vi "remove_invalid_ROI.vi"(8 "error in (no error)":errorcluster, 9 "number of particles":i32, 10 "Image Pixels in":u8[][](array[numeric]), 11 "SegmenterMG100305SingleCell in":refnum<class "SegmenterMG100305SingleCell.lvclass">) -> (0 "error out":errorcluster, 1 "ROI array out":cluster{"x":i32, "y":i32}[](array[cluster]), 2 "Image Pixels out":u8[][](array[numeric]), 3 "SegmenterMG100305SingleCell out":refnum<class "SegmenterMG100305SingleCell.lvclass">)   [LabVIEW 2010, in "SegmenterMG100305SingleCell.lvclass"]
uses:
  SegmenterMG100305SingleCell.lvclass
  <vilib>/Analysis/Matrix/Datatypes/RealMatrix.ctl
  <vilib>/Analysis/Matrix/NI_Matrix.lvlib
panel:
  out "Real Matrix":T1
  out "Numeric":i32
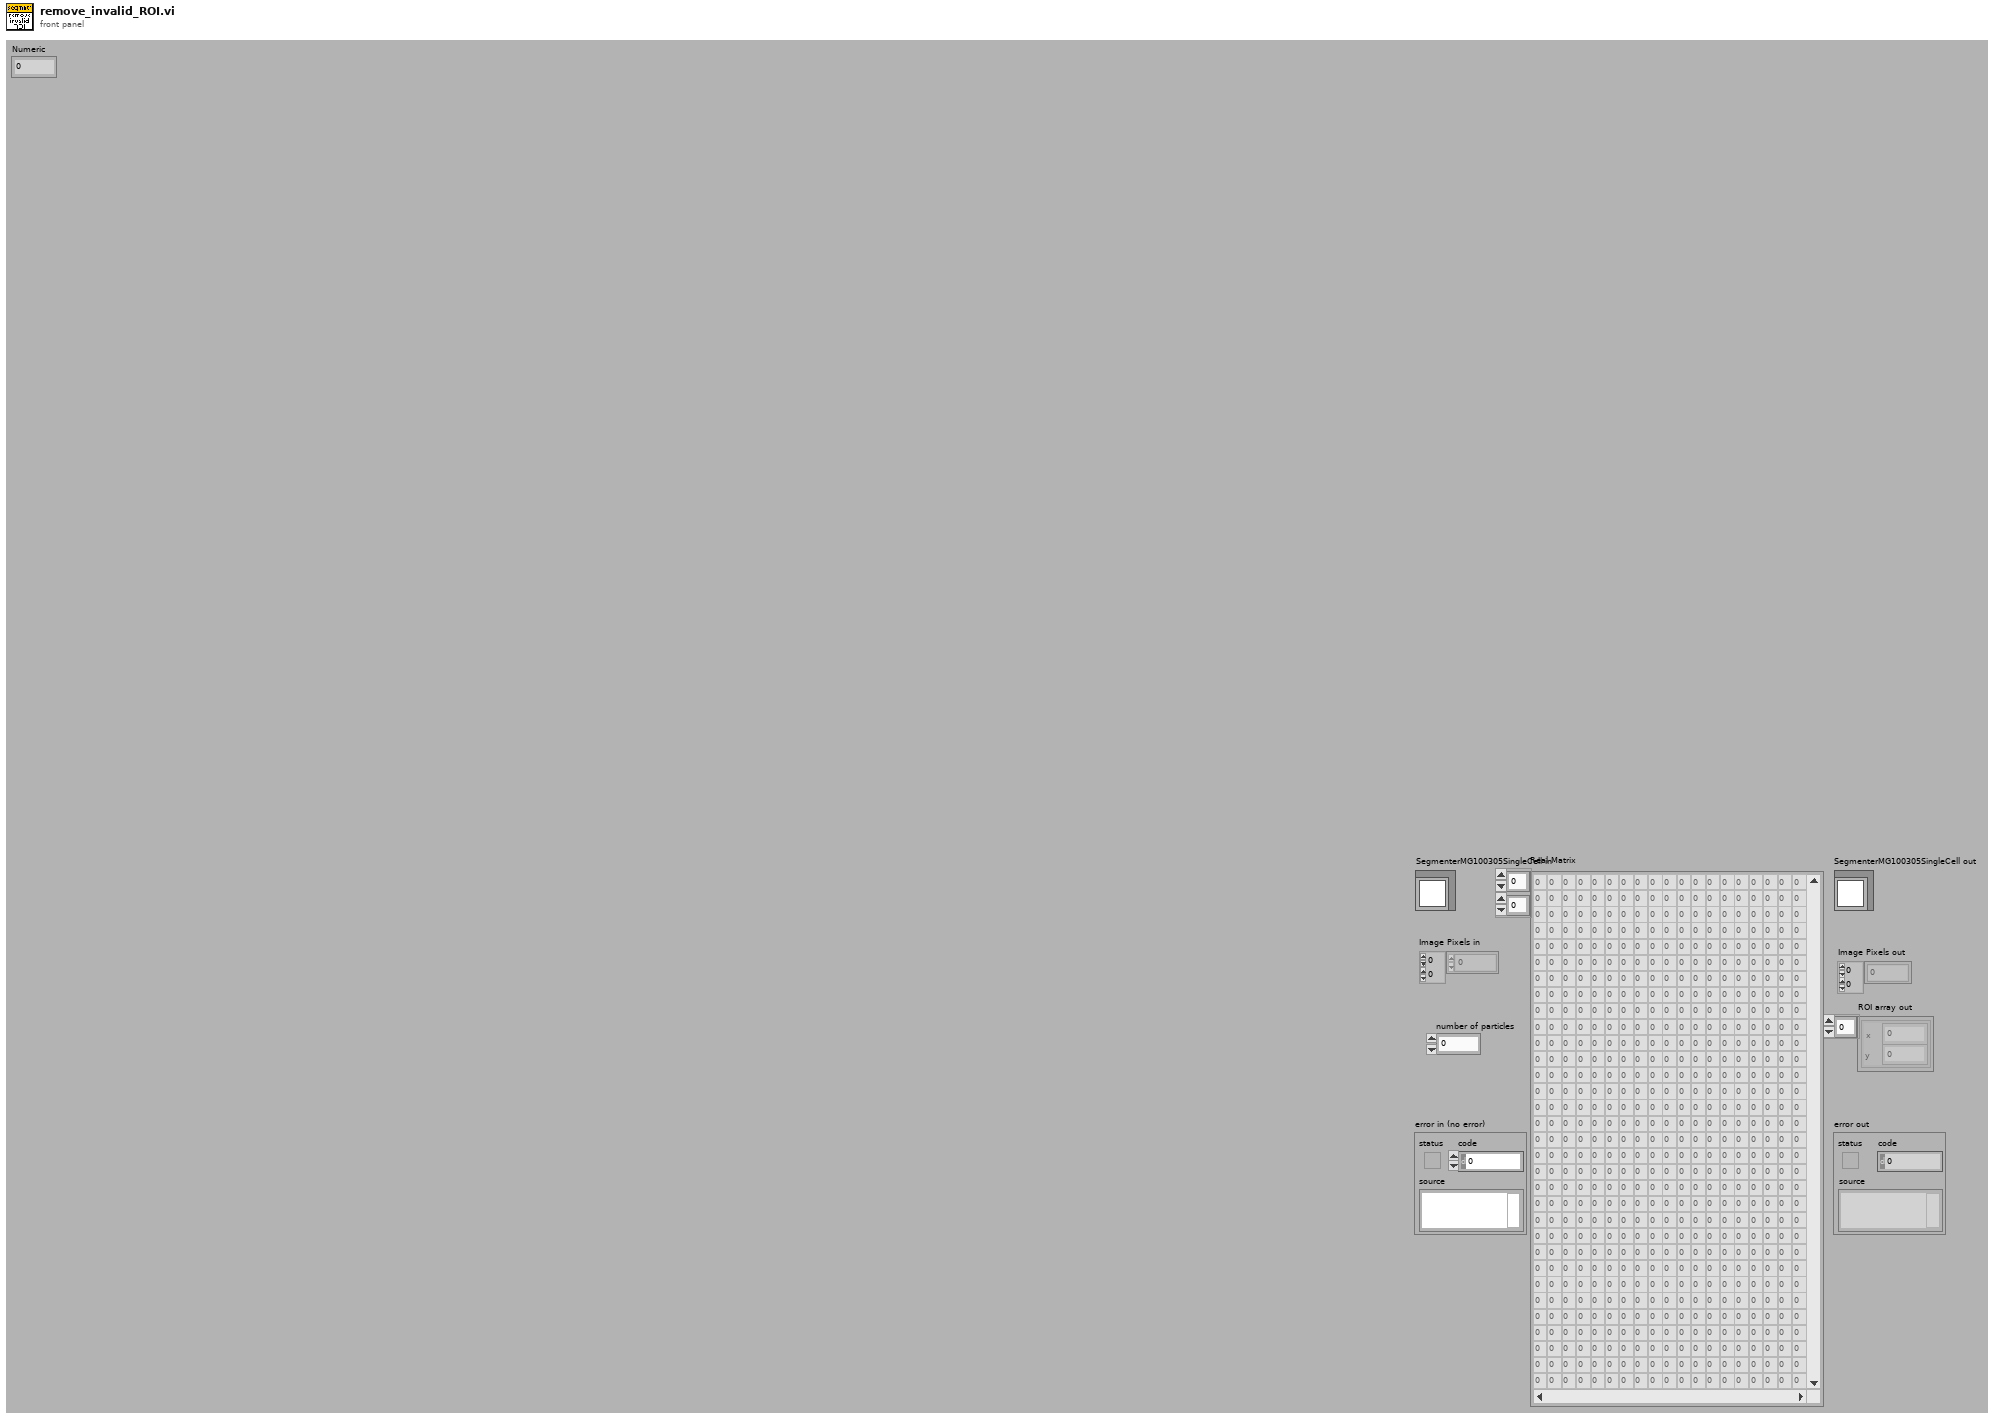
[diagram p1: front panel]
types:
  T1 = typedef "NI_Matrix.lvlib/RealMatrix.ctl" = dbl[][]
  T2 = cluster{"[0]":i32, "[1]":i32, "[2]":i32, "[3]":i32, "[4]":i32, "[5]":i32, "[6]":i32, "[7]":i32, "[8]":i32}
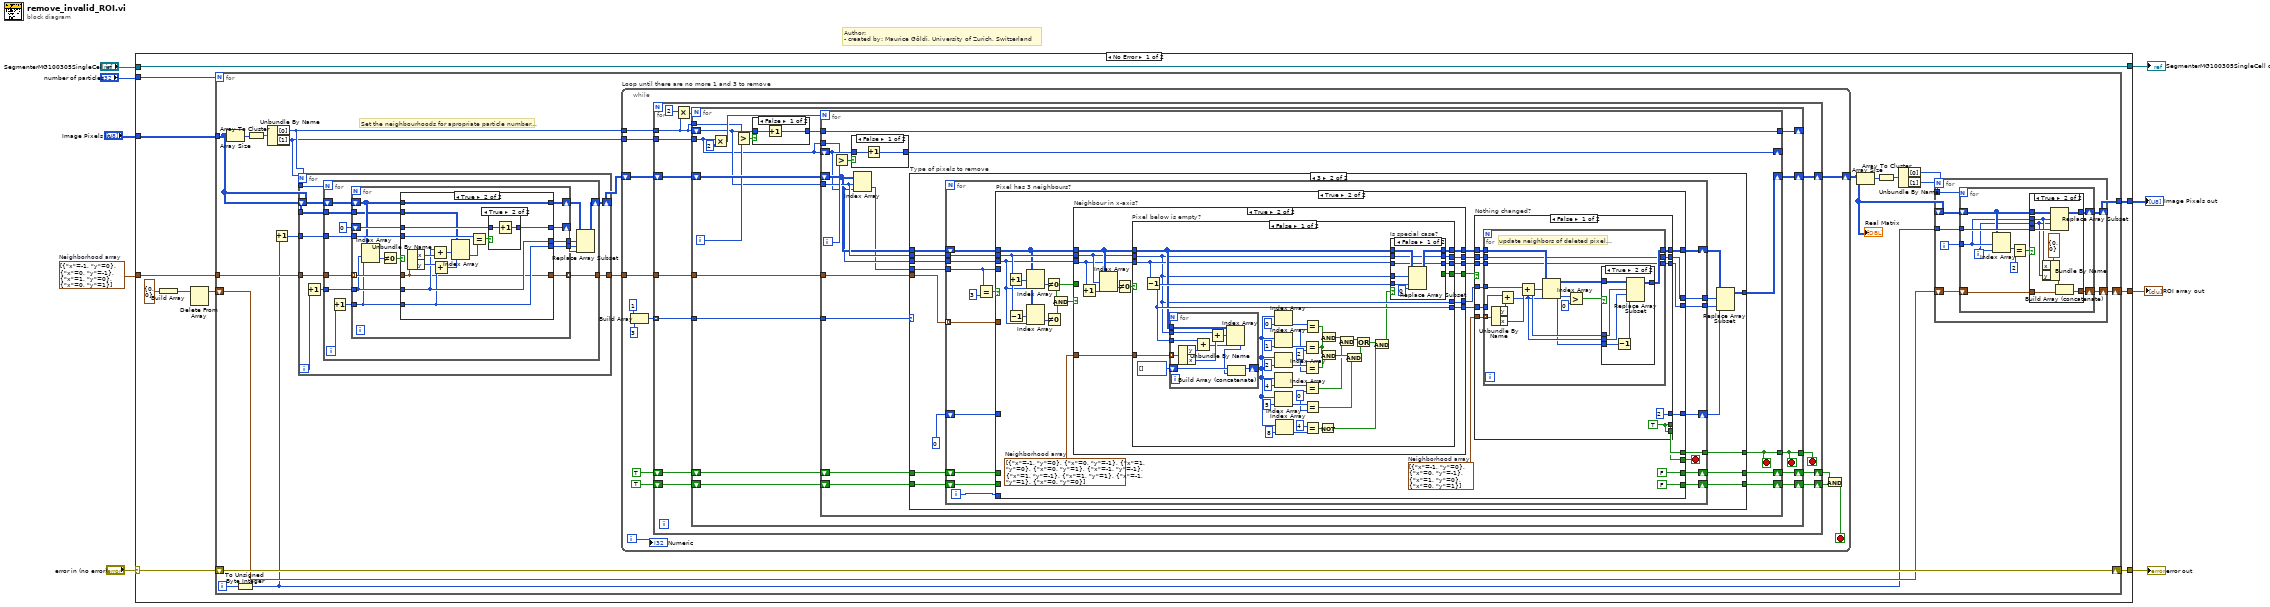
[diagram p0: block diagram]
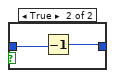
[diagram p5: hidden frame]
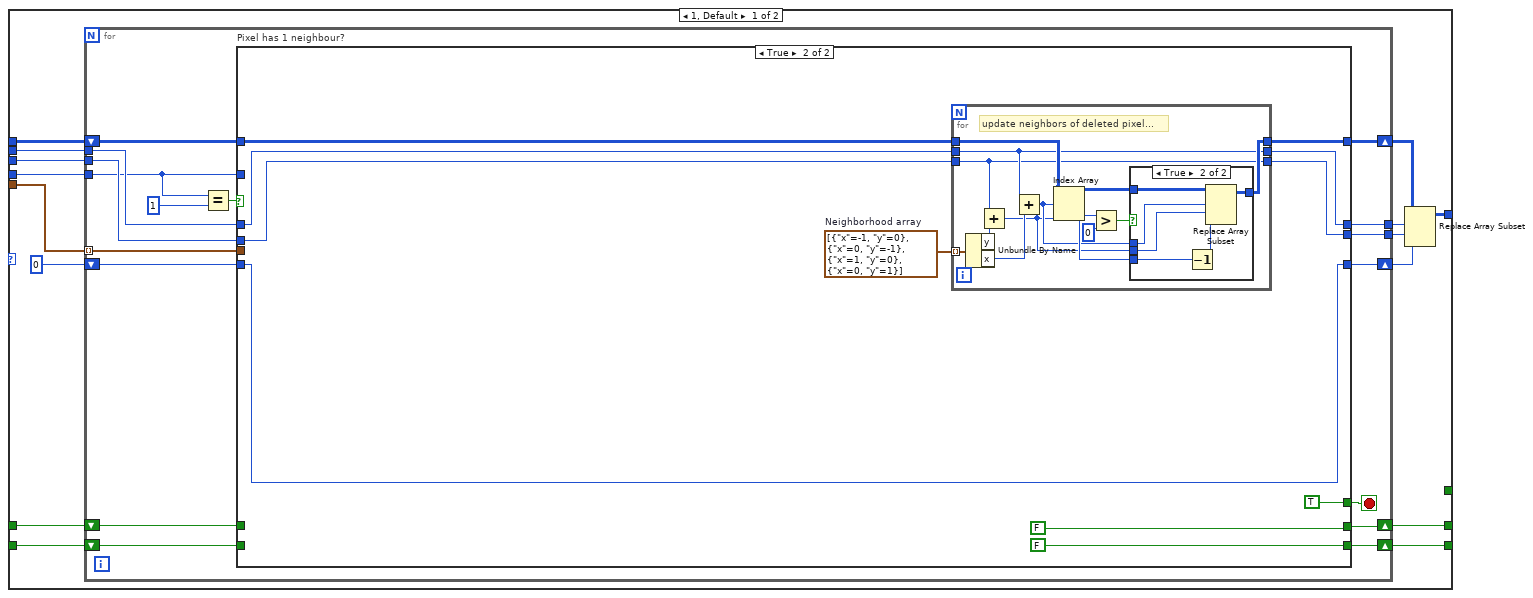
[diagram p6: hidden frame]
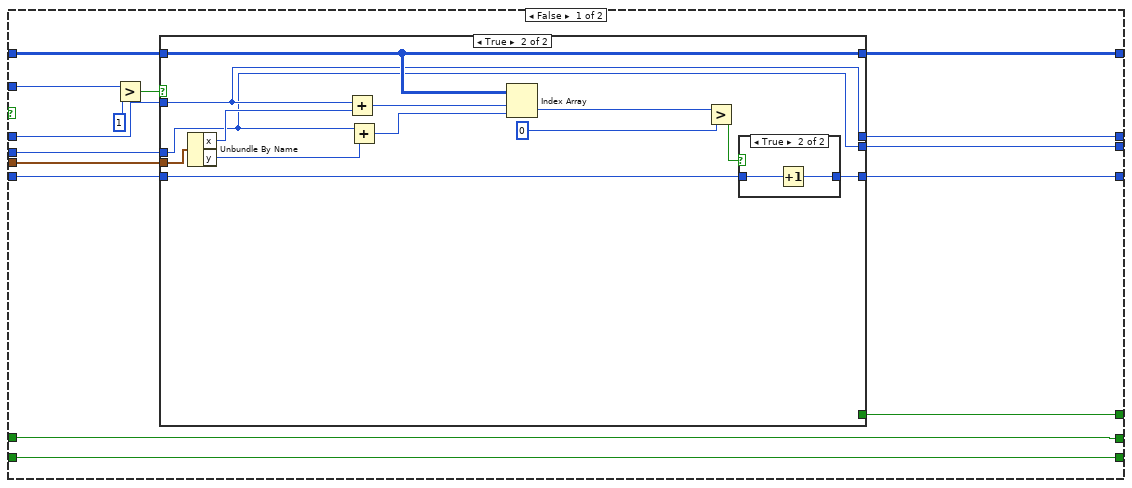
[diagram p7: hidden frame]
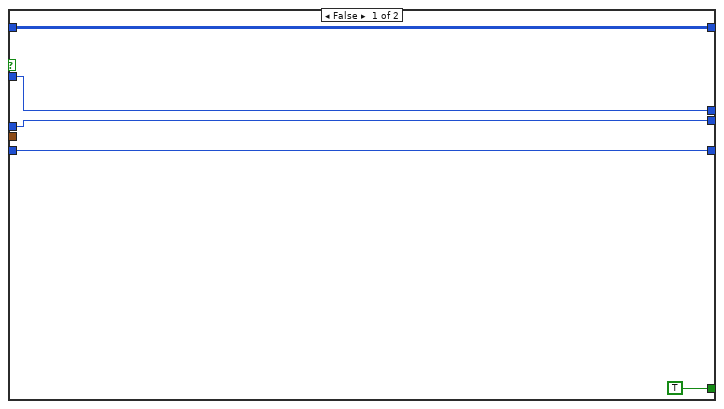
[diagram p8: hidden frame]
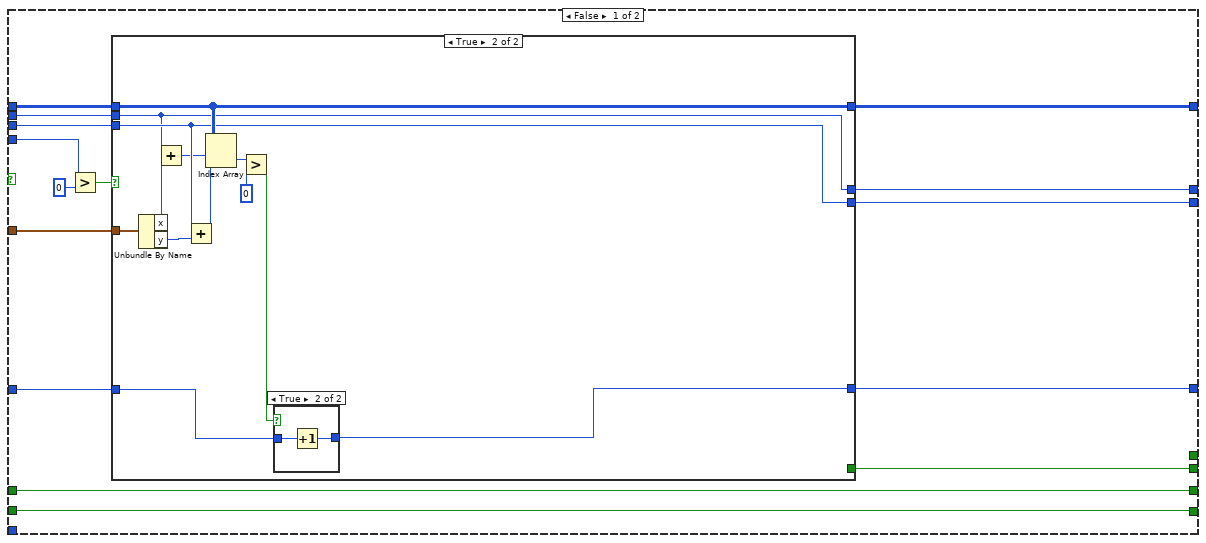
[diagram p11: hidden frame]
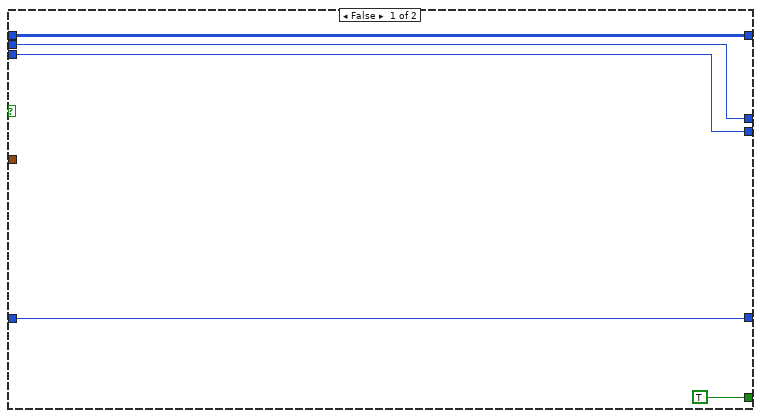
[diagram p12: hidden frame]
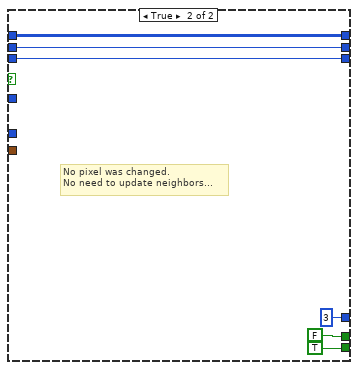
[diagram p15: hidden frame]
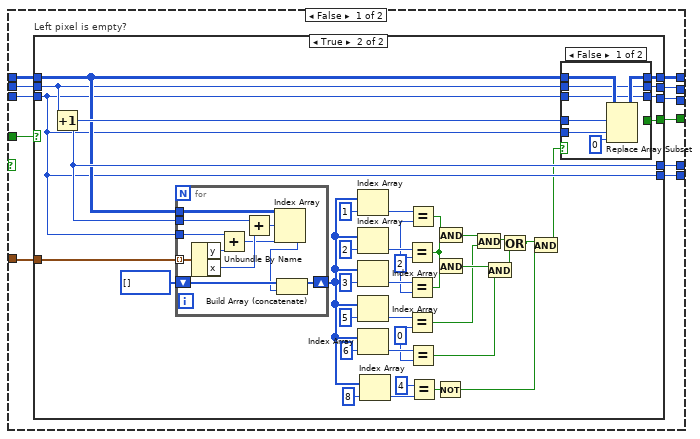
[diagram p16: hidden frame]
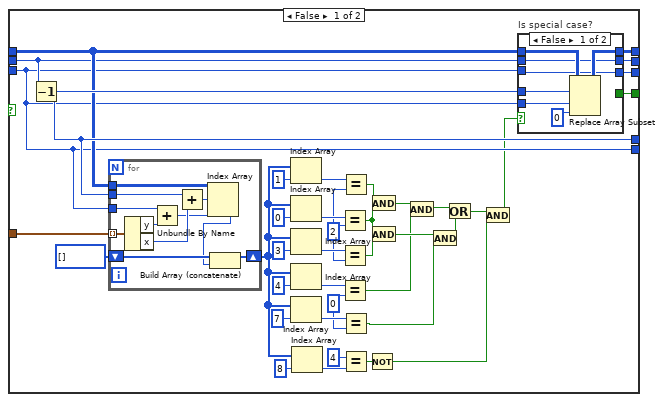
[diagram p17: hidden frame]
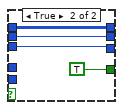
[diagram p18: hidden frame]
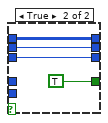
[diagram p19: hidden frame]
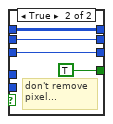
[diagram p20: hidden frame]
diagram:
  w5 = cluster{"x":i32, "y":i32}[] [{"x"=-1, "y"=0}, {"x"=0, "y"=-1}, {"x"=1, "y"=0}, {"x"=0, "y"=1}]  # Neighborhood array
  # "Author: \n- created by: Maurice Göldi, University of Zurich, Switzerland"
  n1 = case shown="No Error" "error in (no error)" {
    selector: "error in (no error)" -> [w17 w700]
    tunnel: [w16 w700] -> w6
    tunnel: "number of particles" -> [w20 _]
    tunnel: "Image Pixels in" -> [w19 _]
    tunnel: w5 -> [w18 _]
    tunnel: [w15 _] -> w1
    tunnel: [w14 _] -> w2
    tunnel: "SegmenterMG100305SingleCell in" -> [w11 w699]
    tunnel: [w11 w699] -> w7
    frame No Error {
      n2 = Build Array(cluster{"x":i32, "y":i32} {"x"=0, "y"=0} ("point")) -> (w13:cluster{"x":i32, "y":i32}[])
      n3 = Delete From Array(array=w13) -> (array with subset deleted=w12:cluster{"x":i32, "y":i32}[])  [unwired: 2 in, 1 out]
      n4 = for {
        N: w20 -> [_]
        tunnel: w19 -> [w22]
        tunnel: w18 -> [w35]
        shift-right: [w40] -> w16
        shift-left: w17 -> [w40]
        shift-right: [w28] -> w15
        shift-left: w12 -> [w27]
        tunnel: [w26] -> w14
        i -> [w25]
        # "Set the neighbourhoods for apropriate particle number..."
        n5 = Array Size(array=w22) -> (size(s)=w39:i32[])
        n6 = To Unsigned Byte Integer(number=w25) -> (unsigned 8bit integer=w24:u8)
        n7 = Array To Cluster(array=w39) -> (cluster=w38:T2)
        n8 = Unbundle By Name(w38) -> ("[0]"=w37:i32, "[1]"=w36:i32)
        n9 = Increment(x=w24) -> (x+1=w33:u8)
        n10 = for {
          N: w37 -> [_]
          tunnel: w36 -> [w77]
          shift-right: [w75] -> w23
          shift-left: w22 -> [w76]
          tunnel: w35 -> [w74]
          tunnel: [w73] -> w34
          tunnel: w33 -> [w70]
          tunnel: w22 -> [w69]
          i -> [w72]
          n11 = Increment(x=w72) -> (x+1=w71:i32)
          n12 = for {
            N: w77 -> [_]
            shift-right: [w82] -> w75
            shift-left: w76 -> [w89]
            tunnel: [w91] -> w73
            tunnel: w74 -> [w90]
            tunnel: w71 -> [w87]
            tunnel: w70 -> [w85]
            tunnel: w69 -> [w78]
            i -> [w88]
            n13 = Increment(x=w88) -> (x+1=w86:i32)
            n14 = for {
              tunnel: [w93] -> w91 mode=indexing
              tunnel: w90 -> [w105] mode=indexing
              shift-right: [w100] -> w83
              shift-left: w89 -> [w98]
              tunnel: w87 -> [w97]
              tunnel: w86 -> [w96]
              tunnel: w85 -> [w99]
              shift-right: [w103] -> w81
              shift-left: u8 0 -> [w104]
              tunnel: [w102] -> w80
              tunnel: [w101] -> w79
              tunnel: w78 -> [w92]
              n15 = Index Array(array=w98, index (row)=w97, index (col)=w96) -> (element=w94:u8)
              n16 = Not Equal To 0?(x=w94) -> (x != 0?=w95:bool)
              n17 = case shown="True" w95 {
                tunnel: w105 -> [w106 w112]
                tunnel: w98 -> [w107 w113]
                tunnel: w99 -> [_ w118]
                tunnel: w104 -> [w108 w117]
                tunnel: [w108 w116] -> w103
                tunnel: w96 -> [w109 w114]
                tunnel: w97 -> [w110 w115]
                tunnel: [w110 w115] -> w102
                tunnel: [w109 w114] -> w101
                tunnel: [w107 w113] -> w100
                tunnel: [w106 w112] -> w93
                tunnel: w92 -> [_ w111]
                frame False {
                }
                frame True {
                  n18 = Unbundle By Name(w112) -> ("x"=w124:i32, "y"=w123:i32)
                  n19 = Add(x=w115, y=w124) -> (x+y=w122:i32)
                  n20 = Add(x=w123, y=w114) -> (x+y=w121:i32)
                  n21 = Index Array(array=w111, index (row)=w122, index (col)=w121) -> (element=w119:u8)
                  n22 = Equal?(x=w118, y=w119) -> (x = y?=w120:bool)
                  n23 = case shown="True" w120 {
                    tunnel: [w125 w127] -> w116
                    tunnel: w117 -> [w125 w126]
                    frame False {
                    }
                    frame True {
                      n24 = Increment(x=w126) -> (x+1=w127:u8)
                    }
                  }
                }
              }
            }
            n25 = Replace Array Subset(array=w83, new element=w81, index (row)=w80, index (col)=w79) -> (w82:u8[][])
          }
        }
        n26 = while "Loop until there are no more 1 and 3 to remove" {
          tunnel: w34 -> [w141]
          tunnel: w37 -> [w136]
          tunnel: w36 -> [w135]
          shift-right: [w134] -> w21
          shift-left: w23 -> [w133]
          i -> [w132]
          stop <- w130 stop-if-true
          n27 = Build Array(1 ("element"), 3 ("element")) -> (w138:i32[])
          n28 = for {
            tunnel: w141 -> [w151]
            tunnel: w138 -> [w150] mode=indexing
            tunnel: w136 -> [w146]
            tunnel: w135 -> [w148]
            shift-right: [w147] -> w134
            shift-left: w133 -> [w154]
            shift-right: [w143] -> w129
            shift-left: TRUE -> [w149]
            shift-right: [w144] -> w128
            shift-left: TRUE -> [w145]
            stop <- w142 stop-if-true
            n29 = Multiply(x=2, y=w146) -> (x*y=w153:i32)
            n30 = for {
              N: w153 -> [_]
              tunnel: w148 -> [w158]
              shift-right: [w170] -> _
              shift-left: w146 -> [w164]
              shift-right: [w168] -> w147
              shift-left: w154 -> [w169]
              tunnel: w151 -> [w163]
              tunnel: w150 -> [w162]
              shift-right: [w160] -> w143
              shift-left: w149 -> [w161]
              tunnel: w146 -> [w159]
              shift-right: [w156] -> w144
              shift-left: w145 -> [w157]
              tunnel: [w155] -> w142
              i -> [w165]
              stop <- w155 stop-if-true
              n31 = Multiply(x=w158, y=2) -> (x*y=w171:i32)
              n32 = Greater?(x=w159, y=w165) -> (0:w166:bool)
              n33 = case shown="False" w166 {
                tunnel: w164 -> [w174 w175]
                tunnel: [w173 w176] -> w167
                frame False {
                  n34 = Increment(x=w174) -> (x+1=w173:i32)
                }
                frame True {
                  n35 = Decrement(x=w175) -> (x-1=w176:i32)
                }
              }
              n36 = for {
                N: w171 -> [_]
                shift-right: [w192] -> _
                shift-left: w158 -> [w185]
                shift-right: [w183] -> w168
                shift-left: w169 -> [w186]
                tunnel: w164 -> [w187]
                tunnel: w163 -> [w189]
                tunnel: w162 -> [w188]
                shift-right: [w181] -> w160
                shift-left: w161 -> [w182]
                tunnel: w158 -> [w180]
                shift-right: [w178] -> w156
                shift-left: w157 -> [w179]
                tunnel: w167 -> [w193]
                tunnel: [w193] -> w170
                tunnel: [w177] -> w155
                i -> [w190]
                stop <- w177 stop-if-true
                n37 = Greater?(x=w180, y=w190) -> (0:w191:bool)
                n38 = case shown="False" w191 {
                  tunnel: w185 -> [w696 w697]
                  tunnel: [w695 w698] -> w192
                  frame False {
                    n39 = Increment(x=w696) -> (x+1=w695:i32)
                  }
                  frame True {
                    n40 = Decrement(x=w697) -> (x-1=w698:i32)
                  }
                }
                n41 = Index Array(array=w186, index (row)=w187, index (col)=w185) -> (element=w184:u8)
                n42 = case "Type of pixels to remove" shown="3" w188 {
                  tunnel: w189 -> [w208 w303]
                  tunnel: w187 -> [w207 w306]
                  tunnel: w185 -> [w206 w305]
                  tunnel: w186 -> [w205 w307]
                  tunnel: w184 -> [w204 w304]
                  tunnel: [w198 w301] -> w183
                  tunnel: w182 -> [w196 w297]
                  tunnel: [w195 w296] -> w181
                  tunnel: w179 -> [w197 w294]
                  tunnel: [w194 w293] -> w178
                  tunnel: [_ w292] -> w177
                  frame 1, Default {
                    n43 = for {
                      tunnel: w208 -> [w219] mode=indexing
                      tunnel: w207 -> [w223]
                      tunnel: w206 -> [w222]
                      shift-right: [w216] -> w201
                      shift-left: w205 -> [w220]
                      tunnel: w204 -> [w221]
                      shift-right: [w217] -> w202
                      shift-left: u8 0 -> [w218]
                      tunnel: [w215] -> w200
                      tunnel: [w214] -> w199
                      shift-right: [w212] -> w194
                      shift-left: w197 -> [w211]
                      shift-right: [w209] -> w195
                      shift-left: w196 -> [w210]
                      stop <- w213 stop-if-true
                      n44 = Equal?(x=w221, y=u8 1) -> (x = y?=w224:bool)
                      n45 = case "Pixel has 1 neighbour?" shown="True" w224 {
                        tunnel: w220 -> [w232 w268]
                        tunnel: w223 -> [w236 w266]
                        tunnel: w222 -> [w235 w265]
                        tunnel: w221 -> [w239 _]
                        tunnel: w219 -> [w237 _]
                        tunnel: w218 -> [w234 w264]
                        tunnel: [w233 w264] -> w217
                        tunnel: [w231 w269] -> w216
                        tunnel: [w230 w263] -> w215
                        tunnel: [w229 w262] -> w214
                        tunnel: [w228 TRUE] -> w213
                        tunnel: [w226 FALSE] -> w212
                        tunnel: w211 -> [w226 _]
                        tunnel: [w227 FALSE] -> w209
                        tunnel: w210 -> [w227 _]
                        frame False {
                          n46 = Greater?(x=w239, y=u8 1) -> (0:w240:bool)
                          n47 = case shown="True" w240 {
                            tunnel: w232 -> [w244 w250]
                            tunnel: w237 -> [_ w256]
                            tunnel: w236 -> [w243 w249]
                            tunnel: w235 -> [w242 w248]
                            tunnel: w234 -> [w245 w252]
                            tunnel: [w245 w251] -> w233
                            tunnel: [w244 w250] -> w231
                            tunnel: [w243 w249] -> w230
                            tunnel: [w242 w248] -> w229
                            tunnel: [TRUE _] -> w228
                            frame False {
                            }
                            frame True {
                              n48 = Unbundle By Name(w256) -> ("x"=w257:i32, "y"=w258:i32)
                              n49 = Add(x=w249, y=w257) -> (x+y=w247:i32)
                              n50 = Add(x=w248, y=w258) -> (x+y=w246:i32)
                              n51 = Index Array(array=w250, index (row)=w247, index (col)=w246) -> (element=w255:u8)
                              n52 = Greater?(x=w255, y=u8 0) -> (0:w253:bool)
                              n53 = case shown="True" w253 {
                                tunnel: w252 -> [w259 w261]
                                tunnel: [w259 w260] -> w251
                                frame False {
                                }
                                frame True {
                                n54 = Increment(x=w261) -> (x+1=w260:u8)
                                }
                              }
                            }
                          }
                        }
                        frame True {
                          w267 = cluster{"x":i32, "y":i32}[] [{"x"=-1, "y"=0}, {"x"=0, "y"=-1}, {"x"=1, "y"=0}, {"x"=0, "y"=1}]  # Neighborhood array
                          n55 = for {
                            tunnel: w267 -> [w284] mode=indexing
                            tunnel: w265 -> [w273]
                            tunnel: w266 -> [w274]
                            tunnel: [w283] -> w269
                            tunnel: w268 -> [w282]
                            tunnel: [w274] -> w263
                            tunnel: [w273] -> w262
                            # "update neighbors of deleted pixel..."
                            n56 = Unbundle By Name(w284) -> ("y"=w281:i32, "x"=w280:i32)
                            n57 = Add(x=w273, y=w281) -> (x+y=w275:i32)
                            n58 = Add(x=w274, y=w280) -> (x+y=w276:i32)
                            n59 = Index Array(array=w282, index (row)=w276, index (col)=w275) -> (element=w277:u8)
                            n60 = Greater?(x=w277, y=u8 0) -> (0:w279:bool)
                            n61 = case shown="True" w279 {
                              tunnel: [w285 w291] -> w283
                              tunnel: w282 -> [w285 w290]
                              tunnel: w277 -> [_ w287]
                              tunnel: w276 -> [_ w289]
                              tunnel: w275 -> [_ w288]
                              frame False {
                              }
                              frame True {
                                n62 = Decrement(x=w287) -> (x-1=w286:u8)
                                n63 = Replace Array Subset(array=w290, new element=w286, index (row)=w289, index (col)=w288) -> (w291:u8[][])
                              }
                            }
                          }
                        }
                      }
                    }
                    n64 = Replace Array Subset(array=w201, new element=w202, index (row)=w200, index (col)=w199) -> (w198:u8[][])
                  }
                  frame 3 {
                    n65 = for {
                      tunnel: w306 -> [w323]
                      tunnel: w305 -> [w322]
                      tunnel: w304 -> [w314]
                      tunnel: w303 -> [w321] mode=indexing
                      shift-right: [w318] -> w295
                      shift-left: w307 -> [w326]
                      shift-right: [w319] -> w298
                      shift-left: u8 0 -> [w320]
                      tunnel: [w317] -> w300
                      tunnel: [w316] -> w299
                      shift-right: [w312] -> w296
                      shift-left: w297 -> [w313]
                      shift-right: [w310] -> w293
                      shift-left: w294 -> [w311]
                      tunnel: [w309] -> w292
                      i -> [w308]
                      stop <- w315 stop-if-true
                      n66 = Equal?(x=w314, y=u8 3) -> (x = y?=w325:bool)
                      n67 = case "Pixel has 3 neighbours?" shown="True" w325 {
                        tunnel: w326 -> [w339 w378]
                        tunnel: w323 -> [w337 w380]
                        tunnel: w322 -> [w336 w379]
                        tunnel: w321 -> [w338 _]
                        tunnel: w320 -> [w340 _]
                        tunnel: [w341 w364] -> w319
                        tunnel: [w335 w373] -> w318
                        tunnel: [w334 w371] -> w317
                        tunnel: [w333 w370] -> w316
                        tunnel: [w329 w363] -> w315
                        tunnel: w314 -> [w330 _]
                        tunnel: w313 -> [w327 _]
                        tunnel: [w327 FALSE] -> w312
                        tunnel: w311 -> [w328 _]
                        tunnel: [w328 FALSE] -> w310
                        tunnel: [_ w365] -> w309
                        tunnel: w308 -> [_ _]
                        frame False {
                          n68 = Greater?(x=w330, y=u8 0) -> (0:w332:bool)
                          n69 = case shown="True" w332 {
                            tunnel: [w346 w359] -> w341
                            tunnel: w340 -> [w346 w358]
                            tunnel: w339 -> [w342 w355]
                            tunnel: w338 -> [_ w357]
                            tunnel: w337 -> [w344 w348]
                            tunnel: w336 -> [w345 w351]
                            tunnel: [w342 w355] -> w335
                            tunnel: [w345 w351] -> w333
                            tunnel: [w344 w348] -> w334
                            tunnel: [TRUE _] -> w329
                            frame False {
                            }
                            frame True {
                              n70 = Unbundle By Name(w357) -> ("x"=w347:i32, "y"=w356:i32)
                              n71 = Add(x=w348, y=w347) -> (x+y=w350:i32)
                              n72 = Add(x=w351, y=w356) -> (x+y=w349:i32)
                              n73 = Index Array(array=w355, index (row)=w350, index (col)=w349) -> (element=w354:u8)
                              n74 = Greater?(x=w354, y=u8 0) -> (0:w352:bool)
                              n75 = case shown="True" w352 {
                                tunnel: [w360 w362] -> w359
                                tunnel: w358 -> [w360 w361]
                                frame False {
                                }
                                frame True {
                                n76 = Increment(x=w361) -> (x+1=w362:u8)
                                }
                              }
                            }
                          }
                        }
                        frame True {
                          w367 = cluster{"x":i32, "y":i32}[] [{"x"=-1, "y"=0}, {"x"=0, "y"=-1}, {"x"=1, "y"=0}, {"x"=0, "y"=1}, {"x"=-1, "y"=-1}, {"x"=1, "y"=-1}, {"x"=1, "y"=1}, {"x"=-1, "y"=1}, {"x"=0, "y"=0}]  # Neighborhood array
                          w376 = cluster{"x":i32, "y":i32}[] [{"x"=-1, "y"=0}, {"x"=0, "y"=-1}, {"x"=1, "y"=0}, {"x"=0, "y"=1}]  # Neighborhood array
                          n77 = Increment(x=w380) -> (x+1=w385:i32)
                          n78 = Decrement(x=w380) -> (x-1=w386:i32)
                          n79 = Index Array(array=w378, index (row)=w385, index (col)=w379) -> (element=w384:u8)
                          n80 = Index Array(array=w378, index (row)=w386, index (col)=w379) -> (element=w383:u8)
                          n81 = Not Equal To 0?(x=w384) -> (x != 0?=w377:bool)
                          n82 = Not Equal To 0?(x=w383) -> (x != 0?=w382:bool)
                          n83 = And(x=w377, y=w382) -> (x .and. y?=w381:bool)
                          n84 = case "Neighbour in x-axis?" shown="True" w381 {
                            tunnel: w380 -> [w435 w568]
                            tunnel: w379 -> [w434 w567]
                            tunnel: w378 -> [w436 w570]
                            tunnel: [w433 w569] -> w372
                            tunnel: [w432 w566] -> w374
                            tunnel: [w431 w565] -> w375
                            tunnel: w377 -> [w437 _]
                            tunnel: [w430 w563] -> w369
                            tunnel: [w429 w564] -> w368
                            tunnel: w367 -> [w428 w562]
                            tunnel: [w427 w561] -> w366
                            frame False {
                              n85 = case "Left pixel is empty?" shown="True" w437 {
                                tunnel: w436 -> [w453 w534]
                                tunnel: w435 -> [w452 w533]
                                tunnel: w434 -> [w449 w531]
                                tunnel: [w476 w537] -> w433
                                tunnel: [w451 w532] -> w432
                                tunnel: [w450 w530] -> w431
                                tunnel: [w449 w531] -> w429
                                tunnel: [w454 w535] -> w430
                                tunnel: w428 -> [w455 w536]
                                tunnel: [w448 w529] -> w427
                                frame False {
                                w463 = u8 0 ("y")
                                w464 = u8 2 ("y")
                                n86 = Decrement(x=w452) -> (x-1=w454:i32)
                                n87 = for {
                                tunnel: w455 -> [w498] mode=indexing
                                tunnel: w449 -> [w496]
                                tunnel: w454 -> [w495]
                                tunnel: w453 -> [w492]
                                shift-right: [w489] -> w443
                                shift-left: u8[] [] -> [w490]
                                n88 = Unbundle By Name(w498) -> ("y"=w497:i32, "x"=w494:i32)
                                n89 = Add(x=w496, y=w497) -> (x+y=w491:i32)
                                n90 = Add(x=w495, y=w494) -> (x+y=w493:i32)
                                n91 = Index Array(array=w492, index (row)=w493, index (col)=w491) -> (element=w488:u8)
                                n92 = Build Array (concatenate)(w490, w488) -> (w489:u8[])
                                }
                                n93 = Index Array(array=w443, index=1) -> (element=w469:u8)
                                n94 = Index Array(array=w443, index=0) -> (element=w468:u8)
                                n95 = Index Array(array=w443, index=3) -> (element=w467:u8)
                                n96 = Index Array(array=w443, index=4) -> (element=w466:u8)
                                n97 = Index Array(array=w443, index=7) -> (element=w465:u8)
                                n98 = Index Array(array=w443, index=8) -> (element=w446:u8)
                                n99 = Equal?(x=w468, y=w464) -> (x = y?=w460:bool)
                                n100 = Equal?(x=w467, y=w464) -> (x = y?=w459:bool)
                                n101 = Equal?(x=w466, y=w463) -> (x = y?=w438:bool)
                                n102 = Equal?(x=w469, y=w464) -> (x = y?=w462:bool)
                                n103 = Equal?(x=w465, y=w463) -> (x = y?=w439:bool)
                                n104 = Equal?(x=u8 4, y=w446) -> (x = y?=w444:bool)
                                n105 = Not(x=w444) -> (.not. x?=w441:bool)
                                n106 = And(x=w462, y=w460) -> (x .and. y?=w461:bool)
                                n107 = And(x=w460, y=w459) -> (x .and. y?=w458:bool)
                                n108 = And(x=w461, y=w438) -> (x .and. y?=w456:bool)
                                n109 = And(x=w458, y=w439) -> (x .and. y?=w457:bool)
                                n110 = Or(x=w456, y=w457) -> (x .or. y?=w442:bool)
                                n111 = And(x=w442, y=w441) -> (x .and. y?=w440:bool)
                                n112 = case "Is special case?" shown="False" w440 {
                                tunnel: [w482 w487] -> w476
                                tunnel: w449 -> [w481 _]
                                tunnel: w454 -> [w480 _]
                                tunnel: w453 -> [w479 w487]
                                tunnel: w452 -> [w478 w486]
                                tunnel: [w478 w486] -> w451
                                tunnel: [w477 w485] -> w450
                                tunnel: w449 -> [w477 w485]
                                tunnel: [_ TRUE] -> w448
                                frame False {
                                n113 = Replace Array Subset(array=w479, new element=u8 0 ("new element/subarray"), index (row)=w480, index (col)=w481) -> (w482:u8[][])
                                }
                                frame True {
                                }
                                }
                                }
                                frame True {
                                w516 = u8 0 ("y")
                                w517 = u8 2 ("y")
                                n114 = Increment(x=w533) -> (x+1=w535:i32)
                                n115 = for {
                                tunnel: w536 -> [w548] mode=indexing
                                tunnel: w531 -> [w546]
                                tunnel: w535 -> [w545]
                                tunnel: w534 -> [w542]
                                shift-right: [w539] -> w508
                                shift-left: u8[] [] -> [w540]
                                n116 = Unbundle By Name(w548) -> ("y"=w547:i32, "x"=w544:i32)
                                n117 = Add(x=w546, y=w547) -> (x+y=w541:i32)
                                n118 = Add(x=w545, y=w544) -> (x+y=w543:i32)
                                n119 = Index Array(array=w542, index (row)=w543, index (col)=w541) -> (element=w538:u8)
                                n120 = Build Array (concatenate)(w540, w538) -> (w539:u8[])
                                }
                                n121 = Index Array(array=w508, index=1) -> (element=w522:u8)
                                n122 = Index Array(array=w508, index=2) -> (element=w521:u8)
                                n123 = Index Array(array=w508, index=3) -> (element=w520:u8)
                                n124 = Index Array(array=w508, index=5) -> (element=w519:u8)
                                n125 = Index Array(array=w508, index=6) -> (element=w518:u8)
                                n126 = Index Array(array=w508, index=8) -> (element=w506:u8)
                                n127 = Equal?(x=w521, y=w517) -> (x = y?=w513:bool)
                                n128 = Equal?(x=w520, y=w517) -> (x = y?=w512:bool)
                                n129 = Equal?(x=w519, y=w516) -> (x = y?=w499:bool)
                                n130 = Equal?(x=w522, y=w517) -> (x = y?=w515:bool)
                                n131 = Equal?(x=w518, y=w516) -> (x = y?=w500:bool)
                                n132 = Equal?(x=u8 4, y=w506) -> (x = y?=w504:bool)
                                n133 = Not(x=w504) -> (.not. x?=w501:bool)
                                n134 = And(x=w515, y=w513) -> (x .and. y?=w514:bool)
                                n135 = And(x=w513, y=w512) -> (x .and. y?=w511:bool)
                                n136 = And(x=w514, y=w499) -> (x .and. y?=w509:bool)
                                n137 = And(x=w511, y=w500) -> (x .and. y?=w510:bool)
                                n138 = Or(x=w509, y=w510) -> (x .or. y?=w502:bool)
                                n139 = And(x=w502, y=w501) -> (x .and. y?=w503:bool)
                                n140 = case shown="False" w503 {
                                tunnel: [w555 w559] -> w537
                                tunnel: w535 -> [w553 _]
                                tunnel: w531 -> [w552 _]
                                tunnel: w534 -> [w551 w559]
                                tunnel: w533 -> [w550 w558]
                                tunnel: [w550 w558] -> w532
                                tunnel: w531 -> [w549 w557]
                                tunnel: [w549 w557] -> w530
                                tunnel: [_ TRUE] -> w529
                                frame False {
                                n141 = Replace Array Subset(array=w551, new element=u8 0 ("new element/subarray"), index (row)=w553, index (col)=w552) -> (w555:u8[][])
                                }
                                frame True {
                                }
                                }
                                }
                              }
                            }
                            frame True {
                              n142 = Increment(x=w567) -> (x+1=w572:i32)
                              n143 = Index Array(array=w570, index (row)=w568, index (col)=w572) -> (element=w560:u8)
                              n144 = Not Equal To 0?(x=w560) -> (x != 0?=w571:bool)
                              n145 = case "Pixel below is empty?" shown="False" w571 {
                                tunnel: w570 -> [w608 w649]
                                tunnel: [w611 w672] -> w569
                                tunnel: [w584 w647] -> w566
                                tunnel: w568 -> [w585 w648]
                                tunnel: [w587 w646] -> w565
                                tunnel: w567 -> [w586 w645]
                                tunnel: [w585 w648] -> w563
                                tunnel: [w609 w651] -> w564
                                tunnel: w562 -> [w610 w650]
                                tunnel: [w583 w644] -> w561
                                frame False {
                                w595 = u8 0 ("y")
                                w596 = u8 2 ("y")
                                n146 = Decrement(x=w586) -> (x-1=w609:i32)
                                n147 = for {
                                tunnel: w610 -> [w633] mode=indexing
                                tunnel: w609 -> [w631]
                                tunnel: w585 -> [w630]
                                tunnel: w608 -> [w627]
                                shift-right: [w624] -> w578
                                shift-left: u8[] [] -> [w625]
                                n148 = Unbundle By Name(w633) -> ("y"=w632:i32, "x"=w629:i32)
                                n149 = Add(x=w631, y=w632) -> (x+y=w626:i32)
                                n150 = Add(x=w630, y=w629) -> (x+y=w628:i32)
                                n151 = Index Array(array=w627, index (row)=w628, index (col)=w626) -> (element=w623:u8)
                                n152 = Build Array (concatenate)(w625, w623) -> (w624:u8[])
                                }
                                n153 = Index Array(array=w578, index=0) -> (element=w601:u8)
                                n154 = Index Array(array=w578, index=1) -> (element=w600:u8)
                                n155 = Index Array(array=w578, index=2) -> (element=w599:u8)
                                n156 = Index Array(array=w578, index=4) -> (element=w598:u8)
                                n157 = Index Array(array=w578, index=5) -> (element=w597:u8)
                                n158 = Index Array(array=w578, index=8) -> (element=w581:u8)
                                n159 = Equal?(x=w600, y=w596) -> (x = y?=w592:bool)
                                n160 = Equal?(x=w599, y=w596) -> (x = y?=w591:bool)
                                n161 = Equal?(x=w598, y=w595) -> (x = y?=w573:bool)
                                n162 = Equal?(x=w601, y=w596) -> (x = y?=w594:bool)
                                n163 = Equal?(x=w597, y=w595) -> (x = y?=w574:bool)
                                n164 = Equal?(x=u8 4, y=w581) -> (x = y?=w579:bool)
                                n165 = Not(x=w579) -> (.not. x?=w575:bool)
                                n166 = And(x=w594, y=w592) -> (x .and. y?=w593:bool)
                                n167 = And(x=w592, y=w591) -> (x .and. y?=w590:bool)
                                n168 = And(x=w593, y=w573) -> (x .and. y?=w588:bool)
                                n169 = And(x=w590, y=w574) -> (x .and. y?=w589:bool)
                                n170 = Or(x=w588, y=w589) -> (x .or. y?=w577:bool)
                                n171 = And(x=w577, y=w575) -> (x .and. y?=w576:bool)
                                n172 = case "Is special case?" shown="False" w576 {
                                tunnel: [w617 w622] -> w611
                                tunnel: w609 -> [w616 _]
                                tunnel: w585 -> [w615 _]
                                tunnel: w608 -> [w614 w622]
                                tunnel: [w613 w621] -> w587
                                tunnel: w586 -> [w613 w621]
                                tunnel: w585 -> [w612 w620]
                                tunnel: [w612 w620] -> w584
                                tunnel: [_ TRUE] -> w583
                                frame False {
                                n173 = Replace Array Subset(array=w614, new element=u8 0 ("new element/subarray"), index (row)=w615, index (col)=w616) -> (w617:u8[][])
                                }
                                frame True {
                                # "don't remove\npixel..."
                                }
                                }
                                }
                                frame True {
                                w659 = u8 0 ("y")
                                w660 = u8 2 ("y")
                                n174 = Increment(x=w645) -> (x+1=w651:i32)
                                n175 = for {
                                tunnel: w650 -> [w694] mode=indexing
                                tunnel: w651 -> [w692]
                                tunnel: w648 -> [w691]
                                tunnel: w649 -> [w688]
                                shift-right: [w685] -> w639
                                shift-left: u8[] [] -> [w686]
                                n176 = Unbundle By Name(w694) -> ("y"=w693:i32, "x"=w690:i32)
                                n177 = Add(x=w692, y=w693) -> (x+y=w687:i32)
                                n178 = Add(x=w691, y=w690) -> (x+y=w689:i32)
                                n179 = Index Array(array=w688, index (row)=w689, index (col)=w687) -> (element=w684:u8)
                                n180 = Build Array (concatenate)(w686, w684) -> (w685:u8[])
                                }
                                n181 = Index Array(array=w639, index=0) -> (element=w665:u8)
                                n182 = Index Array(array=w639, index=3) -> (element=w664:u8)
                                n183 = Index Array(array=w639, index=2) -> (element=w663:u8)
                                n184 = Index Array(array=w639, index=7) -> (element=w662:u8)
                                n185 = Index Array(array=w639, index=6) -> (element=w661:u8)
                                n186 = Index Array(array=w639, index=8) -> (element=w642:u8)
                                n187 = Equal?(x=w664, y=w660) -> (x = y?=w656:bool)
                                n188 = Equal?(x=w663, y=w660) -> (x = y?=w655:bool)
                                n189 = Equal?(x=w662, y=w659) -> (x = y?=w634:bool)
                                n190 = Equal?(x=w665, y=w660) -> (x = y?=w658:bool)
                                n191 = Equal?(x=w661, y=w659) -> (x = y?=w635:bool)
                                n192 = Equal?(x=u8 4, y=w642) -> (x = y?=w640:bool)
                                n193 = And(x=w658, y=w656) -> (x .and. y?=w657:bool)
                                n194 = And(x=w656, y=w655) -> (x .and. y?=w654:bool)
                                n195 = Not(x=w640) -> (.not. x?=w637:bool)
                                n196 = And(x=w657, y=w634) -> (x .and. y?=w652:bool)
                                n197 = And(x=w654, y=w635) -> (x .and. y?=w653:bool)
                                n198 = Or(x=w652, y=w653) -> (x .or. y?=w638:bool)
                                n199 = And(x=w638, y=w637) -> (x .and. y?=w636:bool)
                                n200 = case "Is special case?" shown="False" w636 {
                                tunnel: [w679 w681] -> w672
                                tunnel: w651 -> [w677 _]
                                tunnel: w648 -> [w676 _]
                                tunnel: w649 -> [w675 w681]
                                tunnel: w648 -> [w674 w683]
                                tunnel: [w674 w683] -> w647
                                tunnel: [w673 w682] -> w646
                                tunnel: w645 -> [w673 w682]
                                tunnel: [_ TRUE] -> w644
                                frame False {
                                n201 = Replace Array Subset(array=w675, new element=u8 0 ("new element/subarray"), index (row)=w676, index (col)=w677) -> (w679:u8[][])
                                }
                                frame True {
                                # "don't remove\npixel..."
                                }
                                }
                                }
                              }
                            }
                          }
                          n202 = case "Nothing changed?" shown="False" w366 {
                            tunnel: w376 -> [w399 _]
                            tunnel: w375 -> [w398 w424]
                            tunnel: w374 -> [w397 w425]
                            tunnel: [w396 w426] -> w373
                            tunnel: w372 -> [w395 w426]
                            tunnel: [w394 w425] -> w371
                            tunnel: [w393 w424] -> w370
                            tunnel: w369 -> [w392 _]
                            tunnel: w368 -> [w391 _]
                            tunnel: [w389 FALSE] -> w365
                            tunnel: [u8 2 u8 3] -> w364
                            tunnel: [w389 TRUE] -> w363
                            frame False {
                              w389 = TRUE
                              n203 = for {
                                tunnel: w399 -> [w413] mode=indexing
                                tunnel: w398 -> [w409]
                                tunnel: w397 -> [w410]
                                tunnel: [w412] -> w396
                                tunnel: w395 -> [w411]
                                tunnel: [w410] -> w394
                                tunnel: [w409] -> w393
                                tunnel: w392 -> [w403]
                                tunnel: w391 -> [w402]
                                # "update neighbors of deleted pixel..."
                                n204 = Unbundle By Name(w413) -> ("y"=w408:i32, "x"=w407:i32)
                                n205 = Add(x=w402, y=w408) -> (x+y=w404:i32)
                                n206 = Add(x=w403, y=w407) -> (x+y=w405:i32)
                                n207 = Index Array(array=w411, index (row)=w405, index (col)=w404) -> (element=w401:u8)
                                n208 = Greater?(x=w401, y=u8 0) -> (0:w400:bool)
                                n209 = case shown="True" w400 {
                                tunnel: [w414 w420] -> w412
                                tunnel: w411 -> [w414 w419]
                                tunnel: w401 -> [_ w416]
                                tunnel: w405 -> [_ w418]
                                tunnel: w404 -> [_ w417]
                                frame False {
                                }
                                frame True {
                                n210 = Decrement(x=w416) -> (x-1=w415:u8)
                                n211 = Replace Array Subset(array=w419, new element=w415, index (row)=w418, index (col)=w417) -> (w420:u8[][])
                                }
                                }
                              }
                            }
                            frame True {
                              # "No pixel was changed. \nNo need to update neighbors..."
                            }
                          }
                        }
                      }
                    }
                    n212 = Replace Array Subset(array=w295, new element=w298, index (row)=w300, index (col)=w299) -> (w301:u8[][])
                  }
                }
              }
            }
          }
          n213 = And(x=w129, y=w128) -> (x .and. y?=w130:bool)
          "Numeric" <- w132
        }
        "Real Matrix" <- w21
        n214 = Array Size(array=w21) -> (size(s)=w32:i32[])
        n215 = Array To Cluster(array=w32) -> (cluster=w31:T2)
        n216 = Unbundle By Name(w31) -> ("[0]"=w30:i32, "[1]"=w29:i32)
        n217 = for {
          N: w30 -> [_]
          tunnel: w29 -> [w47]
          tunnel: w24 -> [w44]
          shift-right: [w45] -> w26
          shift-left: w21 -> [w46]
          shift-right: [w43] -> w28
          shift-left: w27 -> [w42]
          i -> [w41]
          n218 = for {
            N: w47 -> [_]
            shift-right: [w57] -> w45
            shift-left: w46 -> [w54]
            tunnel: w41 -> [w53]
            tunnel: w44 -> [w56]
            shift-right: [w50] -> w43
            shift-left: w42 -> [w49]
            i -> [w48]
            n219 = Index Array(array=w54, index (row)=w53, index (col)=w48) -> (element=w55:u8)
            n220 = Equal?(x=w55, y=u8 2) -> (x = y?=w52:bool)
            n221 = case shown="True" w52 {
              tunnel: w54 -> [w59 w68]
              tunnel: [w59 w67] -> w57
              tunnel: w53 -> [_ w65]
              tunnel: w48 -> [_ w64]
              tunnel: w56 -> [_ w66]
              tunnel: [w58 w63] -> w50
              tunnel: w49 -> [w58 w61]
              frame False {
              }
              frame True {
                n222 = Bundle By Name(cluster=cluster{"x":i32, "y":i32} {"x"=0, "y"=0} ("point"), "x"=w65, "y"=w64) -> (w60:cluster{"x":i32, "y":i32})
                n223 = Replace Array Subset(array=w68, new element=w66, index (row)=w65, index (col)=w64) -> (w67:u8[][])
                n224 = Build Array (concatenate)(w60, w61) -> (w63:cluster{"x":i32, "y":i32}[])
              }
            }
          }
        }
      }
    }
    frame Error {
    }
  }
  "error out" <- w6
  "SegmenterMG100305SingleCell out" <- w7
  "Image Pixels out" <- w2
  "ROI array out" <- w1
